vi "Rumble lister v2.vi"() -> ()   [LabVIEW 2023]
uses:
  <vilib>/Utility/error.llb/Trim Whitespace One-Sided.vi
  <vilib>/Analysis/1siggen.llb/Ramp Pattern by Delta.vi
  <vilib>/httpClient/LabVIEWHTTPClient.lvlib
  <vilib>/Analysis/NI_AALBase.lvlib
panel:
  in  "scan":bool
  in  "kw_case":bool=TRUE
  in  "stop":bool
  in  "Keyword":string caption="Stop on keyword:"
  in  "End time":timestamp=timestamp(3854628000 s since 1904-01-01) format="%<%H:%M %Y-%m-%d>T"
  in  "Start time":timestamp=timestamp(3854624400 s since 1904-01-01) format="%<%H:%M %Y-%m-%d>T"
  in  "scroll":bool=TRUE
  in  "Log file":path
  in  "Threads":i32=4 min=1 max=128
  out "Videos":string
  out "status":string caption="Status"
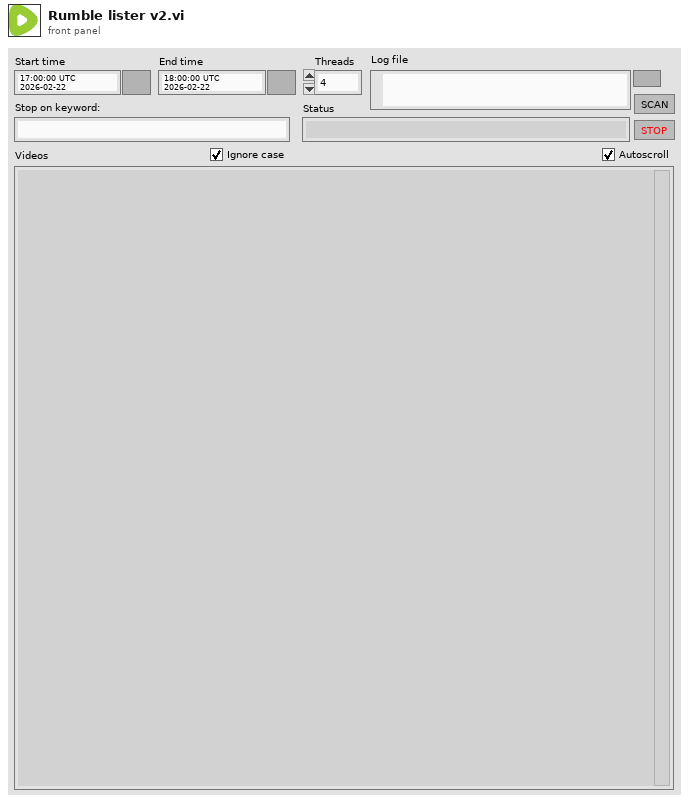
[diagram p1: front panel]
types:
  T1 = cluster{"URL":string, "Video info":string, "HTTP result":i32}
  T2 = enum16{"open", "replace", "create", "open or create", "replace or create", "replace or create with confirmation"}
  T3 = typedef "LabVIEWHTTPClient.lvlib/ClientHandle.ctl" = refnum<k1>
  T4 = cluster{"Video URL":string, "Video info":string, "HTTP result":i32}
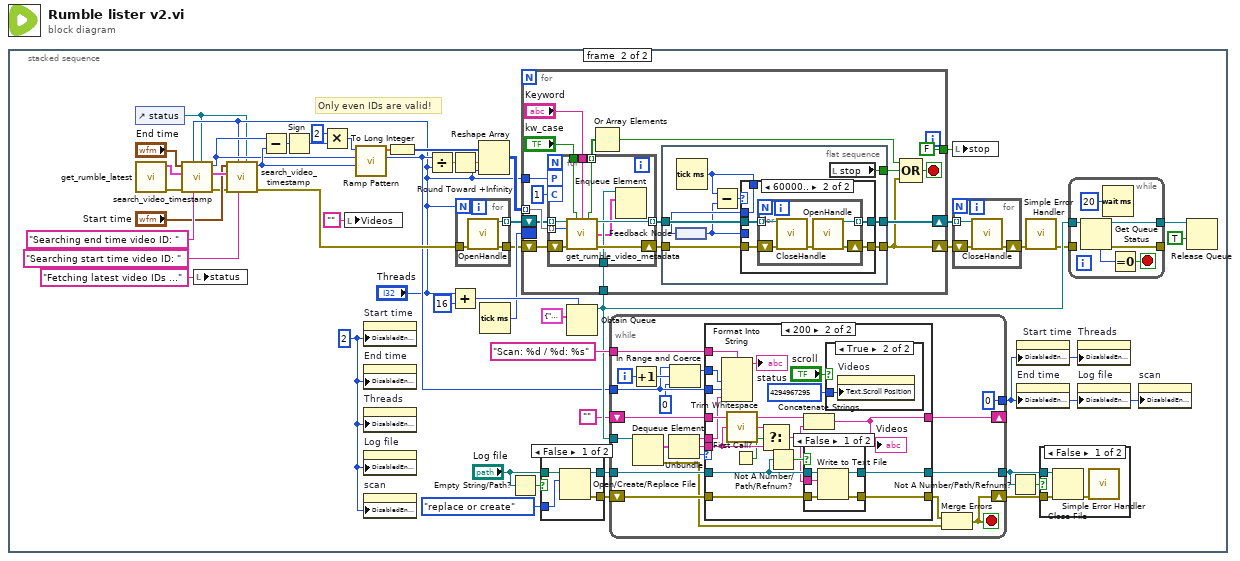
[diagram p0: block diagram]
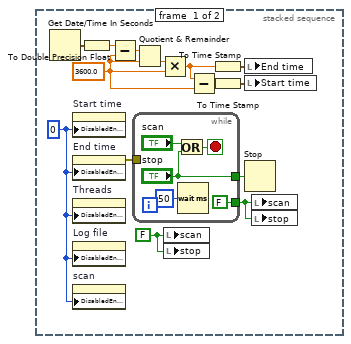
[diagram p2: hidden frame]
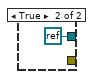
[diagram p4: hidden frame]
diagram:
  n1 = stacked-sequence {
    frame #0 {
      w2 = FALSE
      w5 = u8 0
      w10 = 3600.0 ("y")
      n2 = Get Date/Time In Seconds() -> (seconds since 1Jan1904=w14:timestamp)
      n3 = property on="Start time" class="AbsTime (strict)"("DisabledEnum"=w5) -> ()  [unwired: 2 in, 2 out]
      n4 = property on="End time" class="AbsTime (strict)"("DisabledEnum"=w5) -> (error out=w1:errorcluster)  [unwired: 2 in, 1 out]
      n5 = property on="Threads" class="DigNum (strict)"("DisabledEnum"=w5) -> ()  [unwired: 2 in, 2 out]
      n6 = property on="Log file" class="Path"("DisabledEnum"=w5) -> ()  [unwired: 2 in, 2 out]
      n7 = property on="scan" class="Bool (strict)"("DisabledEnum"=w5) -> ()  [unwired: 2 in, 2 out]
      n8 = To Double Precision Float(number=w14) -> (double precision float=w13:dbl)
      n9 = Subtract(x=w13, y=w10) -> (x-y=w12:dbl)
      n10 = while {
        tunnel: ["stop"] -> w4
        tunnel: [FALSE] -> w3
        tunnel: w1 -> [_]
        stop <- w18 stop-if-true
        n11 = Or(x="scan", y="stop") -> (x .or. y?=w18:bool)
        n12 = Wait (ms)(milliseconds to wait=u32 50) -> ()  [unwired: 1 out]
      }
      n13 = Quotient & Remainder(x=w12, y=w10) -> (floor(x/y)=w11:dbl)  [unwired: 1 out]
      n14 = Multiply(x=w11, y=w10) -> (x*y=w8:dbl)
      n15 = local write "scan"(w2) -> ()
      n16 = local write "stop"(w2) -> ()
      n17 = Subtract(x=w8, y=w10) -> (x-y=w9:dbl)
      n18 = To Time Stamp(1:w8) -> (0:w7:timestamp)
      n19 = To Time Stamp(1:w9) -> (0:w6:timestamp)
      n20 = local write "End time"(w7) -> ()
      n21 = local write "Start time"(w6) -> ()
      n22 = Stop(stop? (T)=w4) -> ()
      n23 = local write "scan"(w3) -> ()
      n24 = local write "stop"(w3) -> ()
    }
    frame #1 {
      w25 = u8 2
      # "Only even IDs are valid!"
      n25 = control-ref of="status"() -> (w20:refnum<vi>)
      n26 = call "get_rumble_latest.vi"() -> ("error out"=w54:errorcluster, "Latest"=w64:cluster{"ID":i32, "Time":timestamp})  [unwired: 9 in, 1 out]
      n27 = call "search_video_timestamp.vi"("Status ref"=w20, "Status prefix"="Searching end time video ID: " ("status"), "Threads (32)"="Threads", "error in (no error)"=w54, "Reference ID record"=w64, "Target time"="End time") -> ("error out"=w56:errorcluster, "ID at target time"=w55:i32)  [unwired: 4 in]
      n28 = local write "status"("Fetching latest video IDs ..." ("status")) -> ()
      n29 = call "search_video_timestamp.vi"("Status ref"=w20, "Status prefix"="Searching start time video ID: " ("status"), "Threads (32)"="Threads", "error in (no error)"=w56, "Reference ID record"=w64, "Target time"="Start time") -> ("error out"=w68:errorcluster, "ID at target time"=w57:i32)  [unwired: 4 in]
      n30 = Subtract(x=w55, y=w57) -> (x-y=w50:i32)
      n31 = Sign(1:w50) -> (0:w58:i32)
      n32 = Multiply(x=2 ("y"), y=w58) -> (x*y=w60:i32)
      n33 = local write "Videos"("") -> ()
      n34 = call-poly <vilib>:"Ramp Pattern.vi"("start"=w57, "end"=w55, "delta"=w60) -> ("samples"=w22:i32, "Ramp Pattern"=w49:dbl[])  [unwired: 6 in, 1 out]
      n35 = property on="Start time" class="AbsTime (strict)"("DisabledEnum"=w25) -> ()  [unwired: 2 in, 2 out]
      n36 = property on="End time" class="AbsTime (strict)"("DisabledEnum"=w25) -> ()  [unwired: 2 in, 2 out]
      n37 = property on="Threads" class="DigNum (strict)"("DisabledEnum"=w25) -> ()  [unwired: 2 in, 2 out]
      n38 = property on="Log file" class="Path"("DisabledEnum"=w25) -> ()  [unwired: 2 in, 2 out]
      n39 = property on="scan" class="Bool (strict)"("DisabledEnum"=w25) -> ()  [unwired: 2 in, 2 out]
      n40 = To Long Integer(number=w49) -> (32bit integer=w61:i32[])
      n41 = Divide(x=w22, y="Threads") -> (x/y=w31:dbl)
      n42 = Round Toward +Infinity(x=w31) -> (ceil(x): smallest int >= x=w32:dbl)
      n43 = Add(x="Threads", y=16) -> (x+y=w52:i32)
      n44 = for {
        N: "Threads" -> [_]
        tunnel: [w138] -> w26 mode=indexing
        tunnel: [w137] -> w27
        tunnel: w68 -> [w136]
        n45 = call <vilib>:"OpenHandle.vi"("error in (no error)"=w136) -> ("client handle out"=w138:T3, "error out"=w137:errorcluster)  [unwired: 13 in]
      }
      n46 = Reshape Array(w61, w32, "Threads") -> (w33:i32[][])
      n47 = Tick Count (ms)() -> (millisecond timer value=w46:u32)
      n48 = Empty String/Path?(string/path="Log file") -> (empty?=w38:bool)
      n49 = case shown="False" w38 {
        tunnel: "Log file" -> [w75 _]
        tunnel: T2."replace or create" ("operation (0:open)") -> [w76 _]
        tunnel: [w74 refnum<k0> refnum] -> w41
        tunnel: [w73 _] -> w42
        frame False {
          n50 = Open/Create/Replace File(file path (use dialog)=w75, operation (0:open)=w76) -> (refnum out=w74:refnum<file>, error out=w73:errorcluster)  [unwired: 4 in, 1 out]
        }
        frame True {
        }
      }
      n51 = Obtain Queue(max queue size (-1, unlimited)=w52, element data type=T1 {"URL"="", "Video info"="", "HTTP result"=0} ("Result")) -> (queue out=w51:refnum<queue>)  [unwired: 3 in, 2 out]
      n52 = for {
        shift-right: [w149] -> w28
        shift-left: w26 -> [w153]
        shift-right: [w148] -> w29
        shift-left: w27 -> [w152]
        tunnel: w33 -> [w154] mode=indexing
        tunnel: "Threads" -> [w145]
        tunnel: w51 -> [w151]
        border: w46 -> [_]
        tunnel: [FALSE] -> w23
        stop <- w155 stop-if-true
        n53 = for {
          tunnel: w154 -> [w183] mode=indexing
          tunnel: w153 -> [w187] mode=indexing
          tunnel: [w185] -> w150 mode=indexing
          tunnel: w151 -> [w182]
          workers-P: w145 -> [_]
          chunk-C: 1 -> [_]
          shift-right: [w184] -> w144
          shift-left: w152 -> [w186]
          tunnel: "kw_case" -> [w180]
          tunnel: "Keyword" -> [w179]
          tunnel: [w178] -> w141 mode=indexing
          n54 = call "get_rumble_video_metadata.vi"("HTTP client handle"=w187, "Keyword ignore case (T)"=w180, "Keyword"=w179, "Video ID"=w183, "error in (no error)"=w186) -> ("Keyword found"=w178:bool, "client handle out"=w185:T3, "Query result"=w181:T4, "error out"=w184:errorcluster)  [unwired: 6 in, 1 out]
          n55 = Enqueue Element(queue=w182, element=w181) -> ()  [unwired: 2 in, 3 out]
        }
        n56 = Or Array Elements(Boolean array=w141) -> (logical OR=w140:bool)
        n57 = flat-sequence {
          tunnel: w150 -> [w163]
          tunnel: w144 -> [w162]
          tunnel: [w161] -> w149
          tunnel: [w160] -> w148
          tunnel: [w156] -> w147
          frame #0 {
            n58 = feedback #1() -> (w157:u32)
            n59 = Tick Count (ms)() -> (millisecond timer value=w159:u32)
            n60 = Subtract(x=w159, y=w157) -> (x-y=w164:u32)
            n61 = case shown="60000.." w164 {
              tunnel: w163 -> [w167 w172]
              tunnel: w162 -> [w166 w171]
              tunnel: [w167 w170] -> w161
              tunnel: [w166 w169] -> w160
              tunnel: [w165 w168] -> w158
              tunnel: w159 -> [_ w168]
              tunnel: w157 -> [w165 _]
              frame Default {
              }
              frame 60000.. {
                n62 = for {
                  tunnel: w172 -> [w177] mode=indexing
                  shift-right: [w173] -> w169
                  shift-left: w171 -> [w176]
                  tunnel: [w174] -> w170 mode=indexing
                  n63 = call <vilib>:"CloseHandle.vi"("client handle"=w177, "error in (no error)"=w176) -> ("error out"=w175:errorcluster)  [unwired: 13 in]
                  n64 = call <vilib>:"OpenHandle.vi"("error in (no error)"=w175) -> ("client handle out"=w174:T3, "error out"=w173:errorcluster)  [unwired: 13 in]
                }
              }
            }
            n65 = feedback-in #1(w158) -> ()
            n66 = local read "stop"() -> (w156:bool)
          }
        }
        n67 = Compound Arithmetic op=OR(w140, w147, w148) -> (w155:bool)
      }
      n68 = while {
        shift-right: [w100] -> _
        shift-left: "" -> [w103]
        tunnel: w51 -> [w102]
        tunnel: w41 -> [w99]
        shift-right: [w91] -> w45
        shift-left: w42 -> [w98]
        tunnel: [w97] -> w44
        tunnel: w22 -> [w86]
        tunnel: "Scan: %d / %d: %s" ("format string") -> [w90]
        tunnel: [u8 0] -> w24
        i -> [w89]
        stop <- w91 stop-if-true
        n69 = Increment(x=w89) -> (x+1=w87:i32)
        n70 = Dequeue Element(queue=w102) -> (element=w101:T1, error out=w92:errorcluster)  [unwired: 2 in, 2 out]
        n71 = Unbundle(w101) -> ("URL"=w94:string, "Video info"=w95:string, "HTTP result"=w96:i32)
        n72 = In Range and Coerce(upper limit=w86, x=w87, lower limit=0) -> (coerced(x)=w85:i32)  [unwired: 1 out]
        n73 = case shown="200" w96 {
          tunnel: w103 -> [w106 w124]
          tunnel: [w106 w123] -> w100
          tunnel: w99 -> [w105 w122]
          tunnel: w98 -> [w104 w121]
          tunnel: [w104 w120] -> w93
          tunnel: [w105 w119] -> w97
          tunnel: w95 -> [_ w110]
          tunnel: w85 -> [_ w115]
          tunnel: w86 -> [_ w114]
          tunnel: w94 -> [_ w113]
          tunnel: w90 -> [_ w111]
          frame Default {
          }
          frame 200 {
            n74 = Format Into String(format string=w111, w115, w114, w113) -> (resulting string=→"status":string)  [unwired: 2 in, 1 out]
            n75 = call <vilib>:"Trim Whitespace.vi"("string"=w110) -> ("trimmed string"=w109:string)  [unwired: 1 in]
            n76 = First Call?() -> (First Call?: T/F=w107:bool)
            n77 = Select(t=w109, s=w107, f=w110) -> (s? t:f=w108:string)
            n78 = Not A Number/Path/Refnum?(number/path/refnum=w122) -> (NaN/Path/Refnum?=w118:bool)
            n79 = Concatenate Strings(w124, w108) -> (w123:string)
            "Videos" <- w123
            n80 = case shown="False" w118 {
              tunnel: w108 -> [w130 _]
              tunnel: w122 -> [w129 w131]
              tunnel: w121 -> [w128 w132]
              tunnel: [w127 w132] -> w120
              tunnel: [w126 w131] -> w119
              frame False {
                n81 = Write to Text File(file (use dialog)=w129, text=w130, error in=w128) -> (refnum out=w126:refnum<file>, error out=w127:errorcluster)  [unwired: 1 in, 1 out]
              }
              frame True {
              }
            }
            n82 = case shown="True" "scroll" {
              tunnel: u32 4294967295 ("Text.Scroll Position") -> [_ w125]
              frame False {
              }
              frame True {
                n83 = property on="Videos" class="Str"("Text.Scroll Position"=w125) -> ()  [unwired: 2 in, 2 out]
              }
            }
          }
        }
        n84 = Merge Errors(w93, w92) -> (w91:errorcluster)
      }
      n85 = local write "stop"(w23) -> ()
      n86 = for {
        tunnel: w28 -> [w135] mode=indexing
        shift-right: [w133] -> w30
        shift-left: w29 -> [w134]
        n87 = call <vilib>:"CloseHandle.vi"("client handle"=w135, "error in (no error)"=w134) -> ("error out"=w133:errorcluster)  [unwired: 13 in]
      }
      n88 = Not A Number/Path/Refnum?(number/path/refnum=w44) -> (NaN/Path/Refnum?=w43:bool)
      n89 = property on="Start time" class="AbsTime (strict)"("DisabledEnum"=w24) -> ()  [unwired: 2 in, 2 out]
      n90 = property on="End time" class="AbsTime (strict)"("DisabledEnum"=w24) -> ()  [unwired: 2 in, 2 out]
      n91 = call <vilib>:"Simple Error Handler.vi"("error in (no error)"=w30) -> ("error out"=w35:errorcluster)  [unwired: 4 in, 4 out]
      n92 = case shown="False" w43 {
        tunnel: w44 -> [w71 _]
        tunnel: w45 -> [w72 _]
        frame False {
          n93 = Close File(refnum=w71, error in=w72) -> (error out=w70:errorcluster)  [unwired: 1 out]
          n94 = call <vilib>:"Simple Error Handler.vi"("error in (no error)"=w70) -> ()  [unwired: 4 in, 5 out]
        }
        frame True {
        }
      }
      n95 = while {
        tunnel: w51 -> [w83]
        tunnel: w35 -> [_]
        tunnel: [w79] -> w36
        tunnel: [w78] -> _
        stop <- w81 stop-if-true
        n96 = Get Queue Status(queue=w83) -> (queue out=w79:refnum<queue>, error out=w78:errorcluster, # elements in queue=w82:i32)  [unwired: 2 in, 5 out]
        n97 = Wait (ms)(milliseconds to wait=u32 20) -> ()  [unwired: 1 out]
        n98 = Equal To 0?(x=w82) -> (x = 0?=w81:bool)
      }
      n99 = property on="Threads" class="DigNum (strict)"("DisabledEnum"=w24) -> ()  [unwired: 2 in, 2 out]
      n100 = property on="Log file" class="Path"("DisabledEnum"=w24) -> ()  [unwired: 2 in, 2 out]
      n101 = property on="scan" class="Bool (strict)"("DisabledEnum"=w24) -> ()  [unwired: 2 in, 2 out]
      n102 = Release Queue(queue=w36, force destroy? (F)=TRUE) -> ()  [unwired: 1 in, 3 out]
    }
  }
